vi "BRig_Host_dataRunState__entryDelete__delDataTS.vi"(4 "output_arrTrials":i32[](array[numeric]), 6 "output_arrTrials_length":i32, 7 "input_idx":i32[](array[numeric]), 8 "output_arrTrials":bool, 9 "input_nTrial":i32, 11 "input_dataTS":u16[][](array[numeric])) -> (3 "output_dataTS":u16[][](array[numeric]), 5 "output_idx":i32[](array[numeric]))   [LabVIEW 2014]
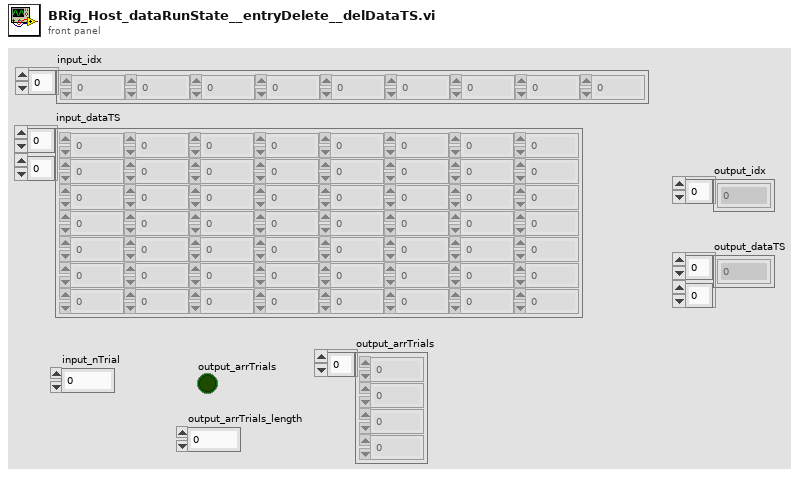
[diagram p1: front panel]
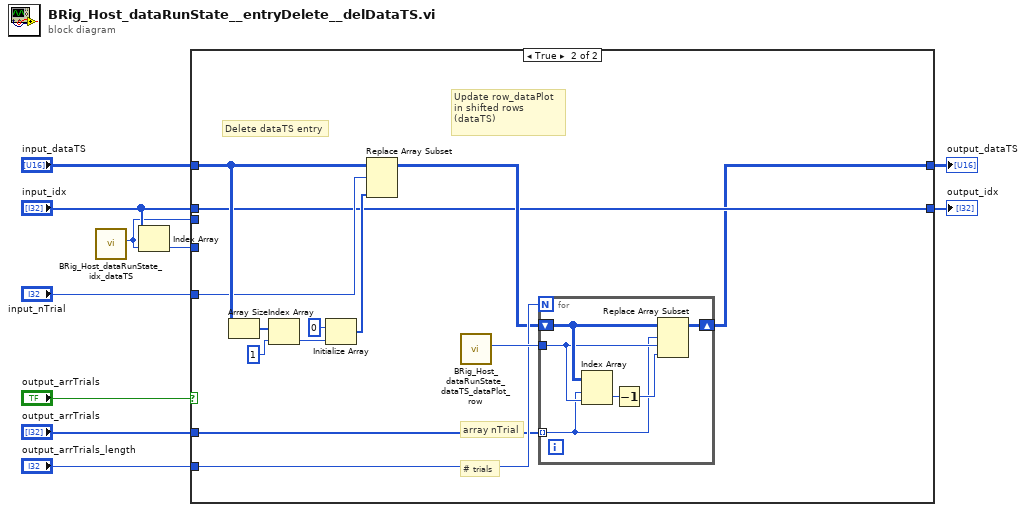
[diagram p0: block diagram]
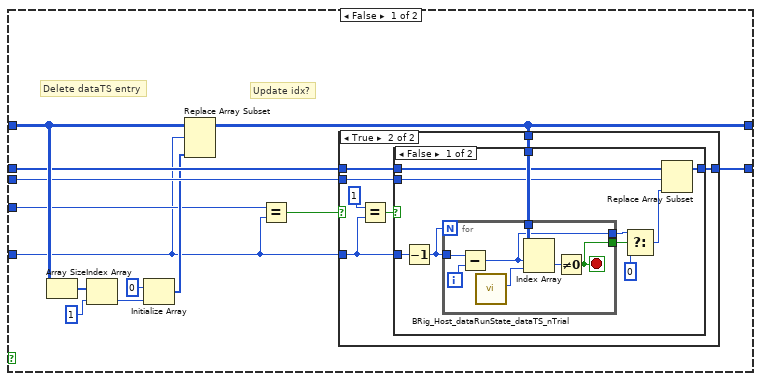
[diagram p2: hidden frame]
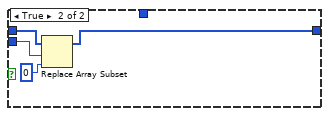
[diagram p4: hidden frame]
diagram:
  n1 = call "BRig_Host_dataRunState_idx_dataTS.vi"() -> ("output_idx_dataTS"=w5:i32)  [unwired: 11 in]
  n2 = Index Array(array="input_idx", index=w5) -> (element=w6:i32)
  n3 = case shown="True" "output_arrTrials" {
    tunnel: "input_idx" -> [w22 w54]
    tunnel: "input_dataTS" -> [w23 w65]
    tunnel: "input_nTrial" -> [w13 w59]
    tunnel: w6 -> [w14 _]
    tunnel: w5 -> [w21 _]
    tunnel: [w11 w53] -> w2
    tunnel: [w20 w54] -> w1
    tunnel: "output_arrTrials" -> [_ w56]
    tunnel: "output_arrTrials_length" -> [_ w57]
    frame False {
      # "Update idx?"
      # "Delete dataTS entry"
      n4 = Array Size(array=w23) -> (size(s)=w19:i32[])
      n5 = Index Array(array=w19, index=1) -> (element=w17:i32)
      n6 = Initialize Array(u16 0 ("element"), w17) -> (w15:u16[])
      n7 = Replace Array Subset(array=w23, new element=w15, index (row)=w13) -> (w11:u16[][])  [unwired: 1 in]
      n8 = Equal?(x=w14, y=w13) -> (x = y?=w12:bool)
      n9 = case shown="True" w12 {
        tunnel: w22 -> [w24 w30]
        tunnel: w21 -> [_ w29]
        tunnel: [w24 w28] -> w20
        tunnel: w13 -> [_ w26]
        tunnel: w11 -> [_ w25]
        frame False {
        }
        frame True {
          n10 = Equal?(x=1 ("y"), y=w26) -> (x = y?=w31:bool)
          n11 = case shown="False" w31 {
            tunnel: w30 -> [w37 w52]
            tunnel: w29 -> [w36 w51]
            tunnel: [w38 w49] -> w28
            tunnel: w26 -> [w41 _]
            tunnel: w25 -> [w39 _]
            frame False {
              n12 = Decrement(x=w41) -> (x-1=w40:i32)
              n13 = for {
                N: w40 -> [_]
                tunnel: w40 -> [w48]
                tunnel: w39 -> [w46]
                tunnel: [w43] -> w35
                tunnel: [w42] -> w34
                i -> [w47]
                stop <- w43 stop-if-true
                n14 = Subtract(x=w48, y=w47) -> (x-y=w42:i32)
                n15 = call "BRig_Host_dataRunState_dataTS_nTrial.vi"() -> ("output_idx_dataTS_nTrial"=w45:i32)  [unwired: 11 in]
                n16 = Index Array(array=w46, index (row)=w42, index (col)=w45) -> (element=w44:u16)
                n17 = Not Equal To 0?(x=w44) -> (x != 0?=w43:bool)
              }
              n18 = Select(t=w34, s=w35, f=0) -> (s? t:f=w32:i32)
              n19 = Replace Array Subset(array=w37, new element=w32, index=w36) -> (w38:i32[])
            }
            frame True {
              n20 = Replace Array Subset(array=w52, new element=0 ("new element/subarray"), index=w51) -> (w49:i32[])
            }
          }
        }
      }
    }
    frame True {
      # "Update row_dataPlot\nin shifted rows\n(dataTS)"
      # "array nTrial"
      # "# trials"
      # "Delete dataTS entry"
      n21 = Array Size(array=w65) -> (size(s)=w64:i32[])
      n22 = Index Array(array=w64, index=1) -> (element=w62:i32)
      n23 = Initialize Array(u16 0 ("element"), w62) -> (w60:u16[])
      n24 = Replace Array Subset(array=w65, new element=w60, index (row)=w59) -> (w55:u16[][])  [unwired: 1 in]
      n25 = call "BRig_Host_dataRunState_dataTS_dataPlot_row.vi"() -> ("output_idx_dataTS_dataPlot_row"=w58:i32)  [unwired: 11 in]
      n26 = for {
        N: w57 -> [_]
        tunnel: w56 -> [w66] mode=indexing
        shift-right: [w70] -> w53
        shift-left: w55 -> [w71]
        tunnel: w58 -> [w69]
        n27 = Index Array(array=w71, index (row)=w66, index (col)=w69) -> (element=w68:u16)
        n28 = Decrement(x=w68) -> (x-1=w67:u16)
        n29 = Replace Array Subset(array=w71, new element=w67, index (row)=w66, index (col)=w69) -> (w70:u16[][])
      }
    }
  }
  "output_dataTS" <- w2
  "output_idx" <- w1
